vi "Teleop.vi"(8 "error in (no error)":errorcluster) -> (0 "error out":errorcluster)   [LabVIEW 2013, in "VirtualRobot.lvlib"]
uses:
  VirtualRobot.lvlib
  <vilib>/ActorFramework/Message Enqueuer/Message Enqueuer.lvclass/Message Enqueuer.ctl
  <vilib>/ActorFramework/Message Enqueuer/Enqueue.vi
  Global Variables.vi
  <vilib>/ActorFramework/Message Priority Queue/Priority Enqueue.vi
  Systems/Driver Messages/Process Teleop Msg/Process Teleop Msg.lvclass
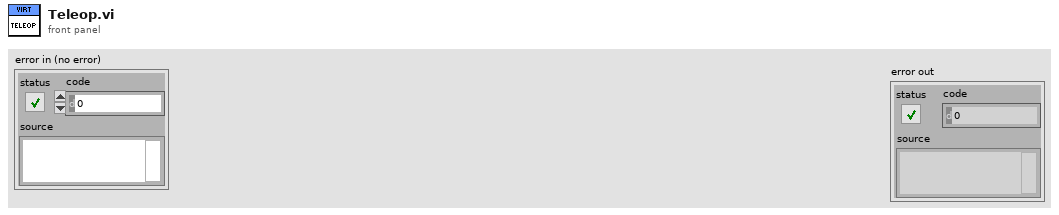
[diagram p1: front panel]
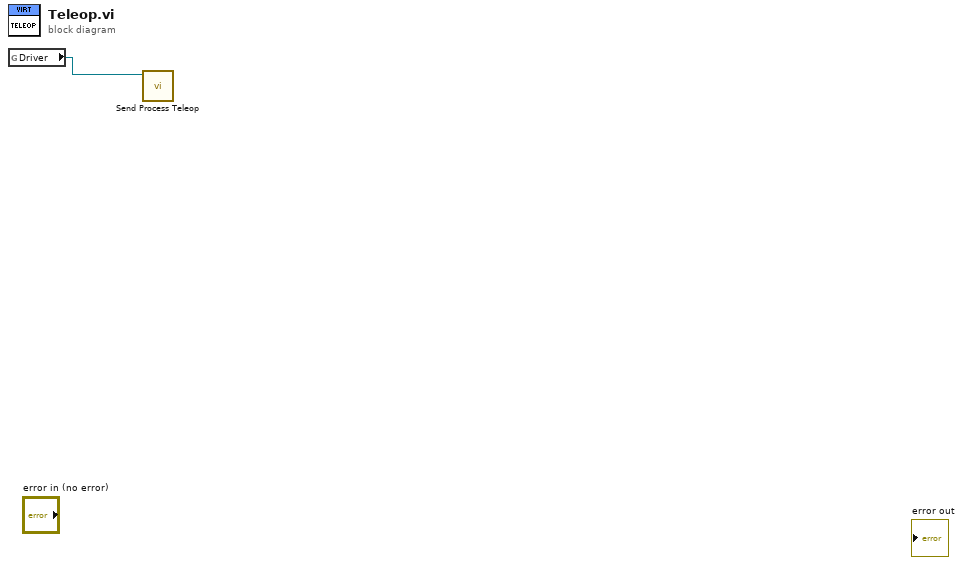
[diagram p0: block diagram]
diagram:
  n1 = global read "Global Variables.vi" "Driver"() -> (w1:refnum<class "Message Enqueuer.lvclass">)
  n2 = call "Send Process Teleop.vi"("Message Enqueuer"=w1) -> ()  [unwired: 9 in, 2 out]
